vi "JKISM++ Request JKISM to Post Message.vi"(6 "Without Reply?(F)":bool, 7 "Module Name":string, 8 "Error In (no error)":errorcluster, 9 "Target Module":string="A", 10 "Arguments (\"\")":string, 11 "State":string="DoA") -> (0 "error out":errorcluster)   [LabVIEW 2014, in "JKI State Machine++.lvlib"]
doc: "Post a message to JKISM specified.\n\n<b>Inputs:</b>\n - <b>Target Module</b>:Target JKISM Module name.\n - <b>State</b>: Message to post.\n - <b>Arguments (\"\")</b>: Argument of the message.\n - <b>Error In (no error)</b>: Error cluster\n\n<b>Outputs:</b>\n - <b>error out</b>: Error cluster"
uses:
  JKI State Machine++.lvlib
  _Support/JKISMQ/_JKISMQFGVOPER.ctl
  _Support/Typedef/_Cross JKISM State Data.ctl
  _Support/Typedef/_JKISM_MSG_TYPE.ctl
  _Support/Typedef/_Cross JKISM State Response.ctl
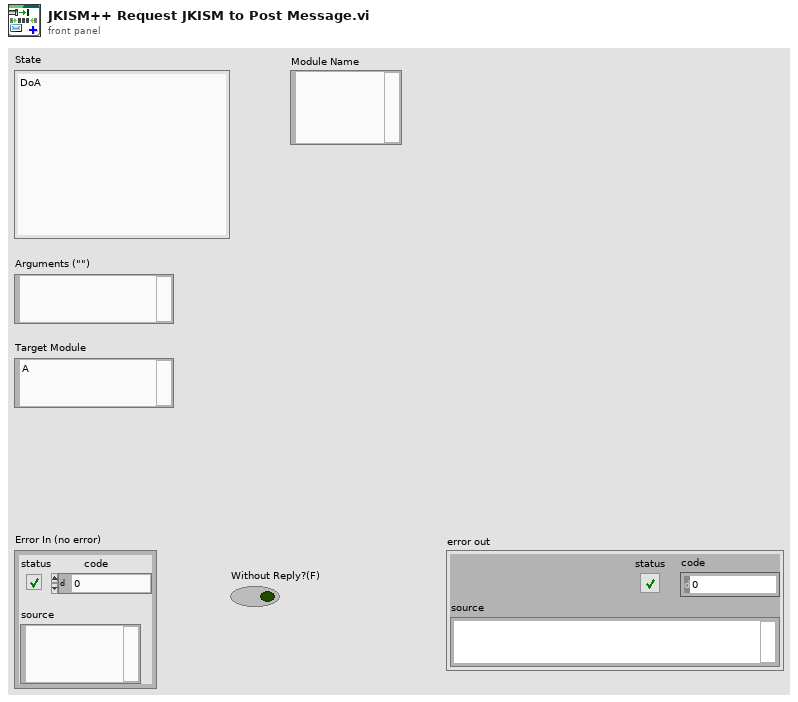
[diagram p1: front panel]
types:
  T1 = typedef "JKI State Machine++.lvlib/_JKISM_MSG_TYPE.ctl" = enum16{"Sync Message(-@)", "Async Message(->)", "Async without Response(->|)", "Async Response", "Broadcast(-><status>)", "Broadcast(-><interrupt>)", "Request to Post Message", "Request to Post Message without Reply", "Request to Publish Status"}
  T2 = typedef "JKI State Machine++.lvlib/_Cross JKISM State Data.ctl" = cluster{"Msg Type":T1, "state":string, "args":string, "source":string, "RespQ":refnum<queue>, "Pre-State":string, "Arg-State":string, "Target":string}
  T3 = typedef "JKI State Machine++.lvlib/_JKISMQFGVOPER.ctl" = enum16{"Get By Name", "List", "Check If Name Exists", "Release", "Module Status"}
  T4 = typedef "JKI State Machine++.lvlib/_JKISMQ.ctl" = cluster{"Module Name":string, "Queue":refnum<queue>, "Locked Status":refnum<data-value>, "Mode":T5, "User Event":refnum<user-event>, "Queue Count":i32}
  T5 = typedef "JKI State Machine++.lvlib/_JKISM_MODE.ctl" = enum16{"Stand Alone", "JKISM", "Action Worker"}
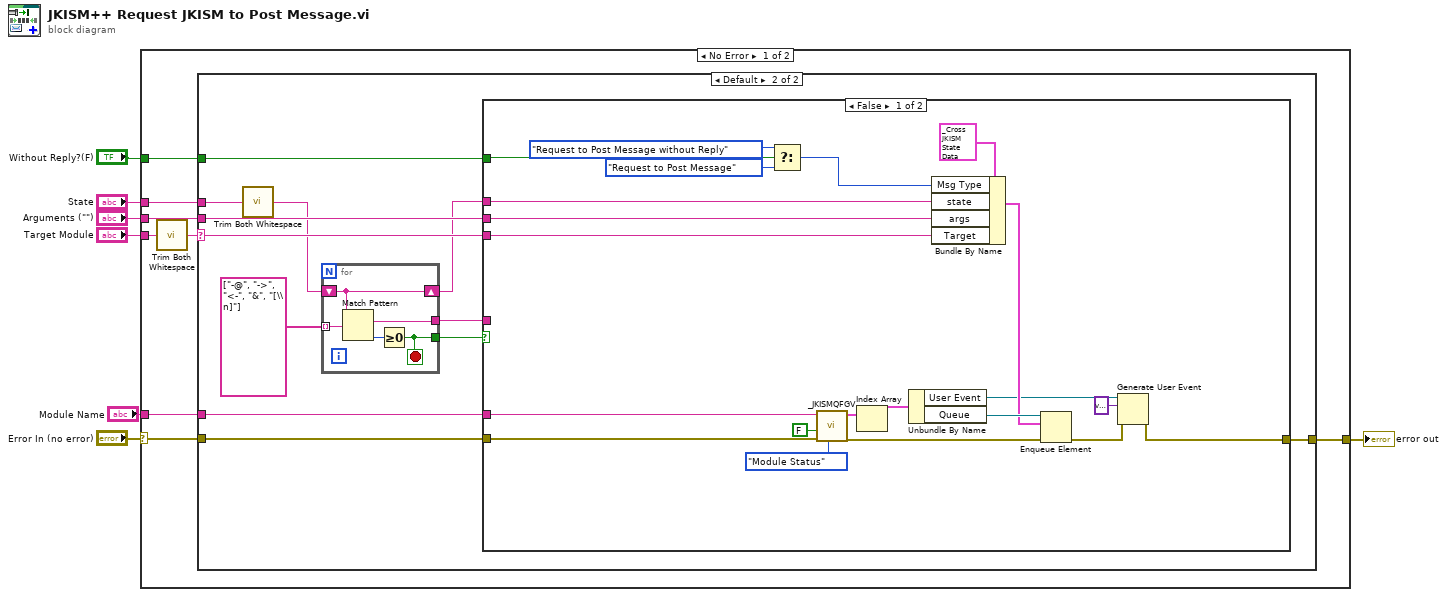
[diagram p0: block diagram]
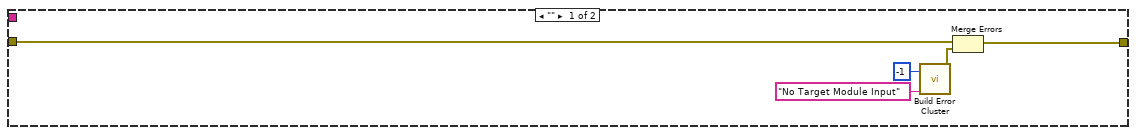
[diagram p2: hidden frame]
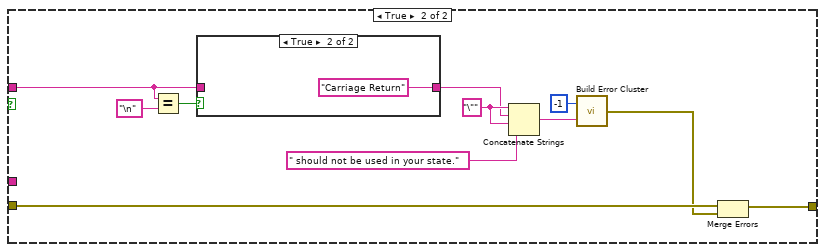
[diagram p3: hidden frame]
diagram:
  n1 = case shown="No Error" "Error In (no error)" {
    selector: "Error In (no error)" -> [w13 w72]
    tunnel: "State" -> [w10 _]
    tunnel: [w14 w72] -> w5
    tunnel: "Arguments (\"\")" -> [w11 _]
    tunnel: "Target Module" -> [w15 _]
    tunnel: "Module Name" -> [w9 _]
    tunnel: "Without Reply?(F)" -> [w8 _]
    frame No Error {
      n2 = call "Trim Both Whitespace.vi"("string"=w15) -> ("trimmed string"=w12:string)  [unwired: 1 in]
      n3 = case shown="Default" w12 {
        selector: w12 -> [_ w31]
        tunnel: w10 -> [_ w27]
        tunnel: w11 -> [_ w32]
        tunnel: [w19 w30] -> w14
        tunnel: w13 -> [w20 w29]
        tunnel: w9 -> [_ w22]
        tunnel: w8 -> [_ w21]
        frame "" {
          n4 = call "Build Error Cluster.vi"("String to Prepend to source (\"\")"="No Target Module Input" ("String to Prepend to source (\"\")"), "code"=-1) -> ("error out"=w18:errorcluster)
          n5 = Merge Errors(w20, w18) -> (w19:errorcluster)
        }
        frame Default {
          n6 = call "Trim Both Whitespace.vi"("string"=w27) -> ("trimmed string"=w23:string)  [unwired: 1 in]
          n7 = for {
            shift-right: [w71] -> w26
            shift-left: w23 -> [w71]
            tunnel: string[] ["-@", "->", "<-", "&", "[\\n]"] -> [w70] mode=indexing
            tunnel: [w68] -> w24
            tunnel: [w67] -> w25
            stop <- w67 stop-if-true
            n8 = Match Pattern(string=w71, regular expression=w70) -> (match substring=w68:string, offset past match=w69:i32)  [unwired: 1 in, 2 out]
            n9 = Greater Or Equal To 0?(x=w69) -> (x >= 0?=w67:bool)
          }
          n10 = case shown="False" w25 {
            tunnel: w32 -> [w46 _]
            tunnel: w31 -> [w45 _]
            tunnel: [w35 w56] -> w30
            tunnel: w29 -> [w43 w57]
            tunnel: w26 -> [w47 _]
            tunnel: w24 -> [_ w54]
            tunnel: w22 -> [w41 _]
            tunnel: w21 -> [w39 _]
            frame False {
              n11 = Select(t=_JKISM_MSG_TYPE."Request to Post Message without Reply" ("Msg Type"), s=w39, f=_JKISM_MSG_TYPE."Request to Post Message" ("Msg Type")) -> (s? t:f=w36:T1)
              n12 = call "_JKISMQFGV.vi"("Operation"=_JKISMQFGVOPER."Module Status", "Error in"=w43, "create if not found? (T)"=FALSE, "Name(\"\" to use uuid) in"=w41) -> ("Error out"=w44:errorcluster, "Array"=w52:T4[])  [unwired: 4 in, 2 out]
              n13 = Index Array(array=w52) -> (element=w51:T4)  [unwired: 1 in]
              n14 = Unbundle By Name(w51) -> ("User Event"=w34:refnum<user-event>, "Queue"=w50:refnum<queue>)
              n15 = Bundle By Name(cluster=T2 {"Msg Type"=enum."Sync Message(-@)", "state"="", "args"="", "source"="", "RespQ"=refnum, "Pre-State"="", "Arg-State"="", "Target"=""} ("element"), "Msg Type"=w36, "state"=w47, "args"=w46, "Target"=w45) -> (w48:T2)
              n16 = Enqueue Element(queue=w50, element=w48, error in (no error)=w44) -> (error out=w42:errorcluster)  [unwired: 1 in, 2 out]
              n17 = Generate User Event(user event=w34, event data cluster=variant ("event data"), error in=w42) -> (error out=w35:errorcluster)  [unwired: 1 in, 1 out]
            }
            frame True {
              w61 = "\"" ("string")
              n18 = Equal?(x=w54, y="\n" ("regular expression")) -> (x = y?=w58:bool)
              n19 = case shown="True" w58 {
                tunnel: [w65 "Carriage Return" ("State")] -> w60
                tunnel: w54 -> [w65 _]
                frame False {
                }
                frame True {
                }
              }
              n20 = Concatenate Strings(w61, w60, w61, " should not be used in your state." ("String to Prepend to source (\"\")")) -> (w62:string)
              n21 = call "Build Error Cluster.vi"("String to Prepend to source (\"\")"=w62, "code"=-1) -> ("error out"=w55:errorcluster)
              n22 = Merge Errors(w57, w55) -> (w56:errorcluster)
            }
          }
        }
      }
    }
    frame Error {
    }
  }
  "error out" <- w5
